vi "Create DI dictionary.vi"(11 "PFI Input":string="/PXI1Slot6/PFI0") -> (3 "map":map{string, string}(c390))   [LabVIEW 2025]
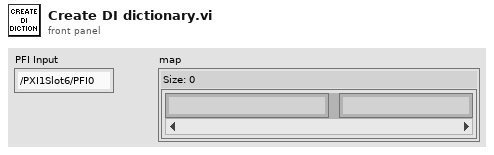
[diagram p1: front panel]
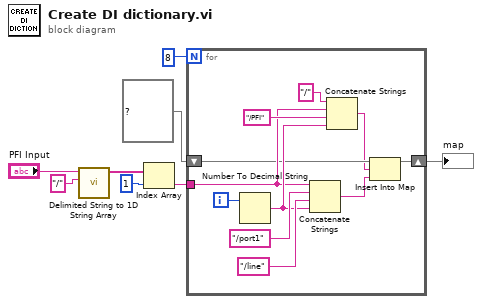
[diagram p0: block diagram]
diagram:
  n1 = call <vilib>:"Delimited String to 1D String Array.vi"("delimiter"="/" ("search string/char (-)"), "delimited string"="PFI Input") -> ("string array"=w6:string[])  [unwired: 9 in]
  n2 = Index Array(array=w6, index=1) -> (element=w3:string)
  n3 = for {
    N: 8 -> [_]
    tunnel: w3 -> [w14]
    shift-right: [w12] -> w1
    shift-left: map{string, string} {} ("map") -> [w11]
    i -> [w19]
    n4 = Number To Decimal String(number=w19) -> (decimal integer string=w15:string)  [unwired: 1 in]
    n5 = Concatenate Strings(w14, "/port1", "/line", w15) -> (w9:string)
    n6 = Concatenate Strings("/" ("string"), w14, "/PFI", w15) -> (w10:string)
    n7 = Insert Into Map(map in=w11, key=w10, value=w9) -> (map out=w12:map{string, string})  [unwired: 2 out]
  }
  "map" <- w1
